vi "Find Spark Wavefronts.vi"(2 "RF Hammer Length":i32, 4 "error in (no error)":errorcluster, 5 "Window Length":i32=10000, 6 "Spark Indicies":i32[](array[numeric]), 7 "Waveform":dbl[](array[numeric])) -> (0 "error out":errorcluster, 1 "Wavefront Indicies":i32[](array[numeric]))   [LabVIEW 2013]
panel:
  out "Waveform Graph":dbl[][](graph)
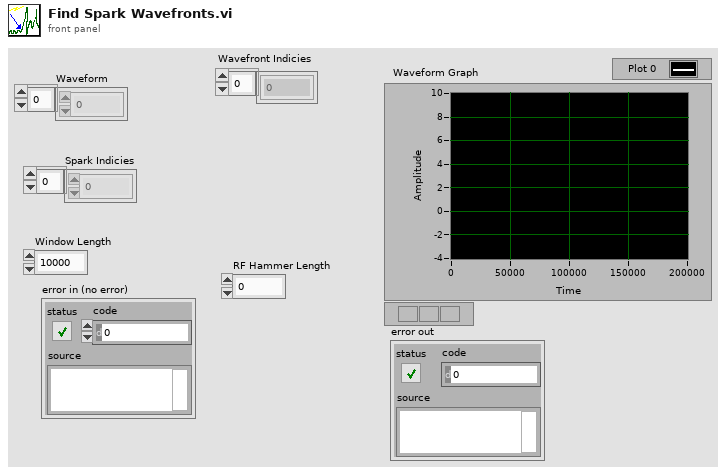
[diagram p1: front panel]
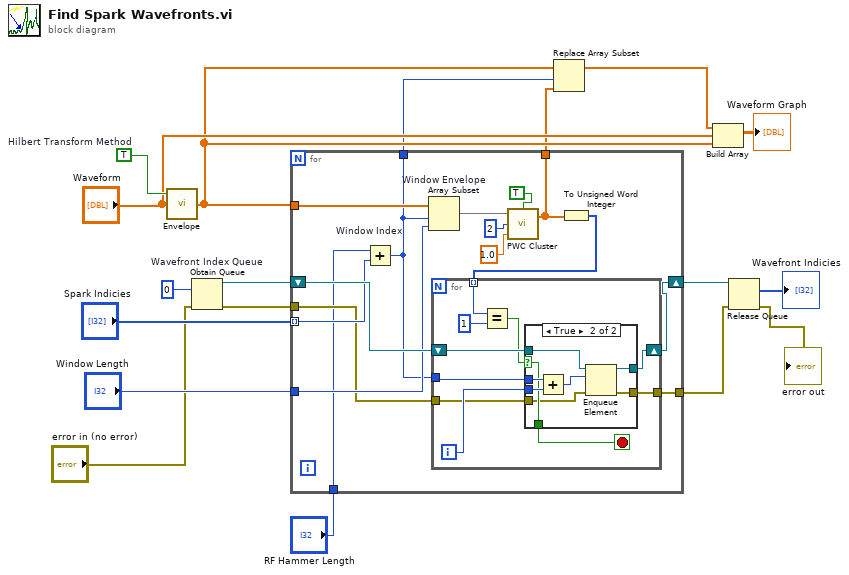
[diagram p0: block diagram]
diagram:
  w6 = TRUE  # Hilbert Transform Method
  n1 = call "Envelope.vi"("Waveform"="Waveform", "Hilbert Transform/Clip Method"=w6) -> ("Envelope"=w4:dbl[])  [unwired: 3 in]
  n2 = Obtain Queue "Wavefront Index Queue"(element data type=0 ("# Cluster Levels"), error in (no error)="error in (no error)") -> (queue out=w18:refnum<queue>, error out=w9:errorcluster)  [unwired: 3 in, 1 out]
  n3 = for {
    tunnel: "Window Length" -> [w28]
    tunnel: "RF Hammer Length" -> [w21]
    tunnel: w4 -> [w30]
    tunnel: "Spark Indicies" -> [w26] mode=indexing
    tunnel: w9 -> [w23]
    tunnel: [w22] -> w8
    tunnel: [w20] -> w3
    tunnel: [w19] -> w2
    shift-right: [w27] -> w16
    shift-left: w18 -> [w29]
    n4 = Add "Window Index"(x=w21, y=w26) -> (x+y=w20:i32)
    n5 = Array Subset "Window Envelope"(array=w30, index=w20, length=w28) -> (w32:dbl[])
    n6 = call "PWC Cluster.vi"("Return Indicies"=TRUE, "Kernel Precission Parameter"=1.0 ("Kernel Parameter/Support"), "# Cluster Levels"=2, "Input Waveform"=w32) -> ("Cluster Assignments"=w19:dbl[])  [unwired: 1 out]
    n7 = To Unsigned Word Integer(number=w19) -> (unsigned 16bit integer=w31:u16[])
    n8 = for {
      tunnel: w31 -> [w43] mode=indexing
      tunnel: w20 -> [w40]
      tunnel: w23 -> [w35]
      tunnel: [w34] -> w22
      shift-right: [w37] -> w27
      shift-left: w29 -> [w42]
      i -> [w41]
      stop <- w38 stop-if-true
      n9 = Equal?(x=w43, y=u16 1) -> (x = y?=w39:bool)
      n10 = case shown="True" w39 {
        selector: w39 -> [w45 w51]
        tunnel: w42 -> [w46 w54]
        tunnel: w41 -> [_ w53]
        tunnel: w40 -> [_ w52]
        tunnel: [w45 w51] -> w38
        tunnel: [w46 w50] -> w37
        tunnel: w35 -> [w44 w48]
        tunnel: [w44 w47] -> w34
        frame False {
        }
        frame True {
          n11 = Add(x=w52, y=w53) -> (x+y=w49:i32)
          n12 = Enqueue Element(queue=w54, element=w49, error in (no error)=w48) -> (queue out=w50:refnum<queue>, error out=w47:errorcluster)  [unwired: 1 in, 1 out]
        }
      }
    }
  }
  n13 = Replace Array Subset(array=w4, new element=w2, index=w3) -> (w1:dbl[])
  n14 = Build Array(w1, "Waveform", w4) -> (→"Waveform Graph":dbl[][])
  n15 = Release Queue(queue=w16, error in (no error)=w8) -> (remaining elements=→"Wavefront Indicies":i32[], error out=→"error out":errorcluster)  [unwired: 1 in, 1 out]
